vi "LabVIEW Measurement UI - Open & Run.vi"(8 "error in":errorcluster, 10 "UI Subpanel":refnum<vi>, 11 "Measurement Client Wrapper in":refnum<class "Measurement Client Wrapper.lvclass">) -> (0 "error out":errorcluster, 2 "Valid UI?":bool, 3 "Measurement Client Wrapper":refnum<class "Measurement Client Wrapper.lvclass">)   [LabVIEW 2020, in "Measurement Client Wrapper.lvclass"]
uses:
  Measurement Client Wrapper.lvclass
  Measurement Client Wrapper.lvclass/Measurement Client Wrapper.ctl
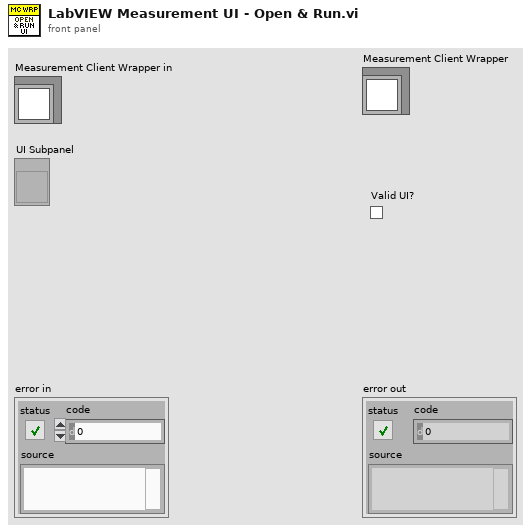
[diagram p1: front panel]
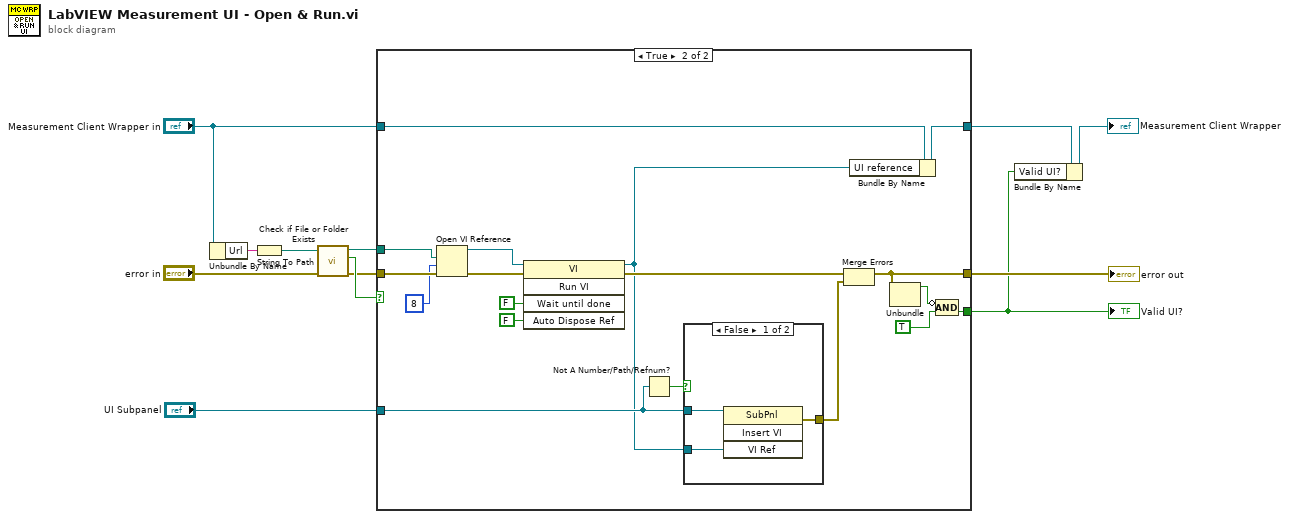
[diagram p0: block diagram]
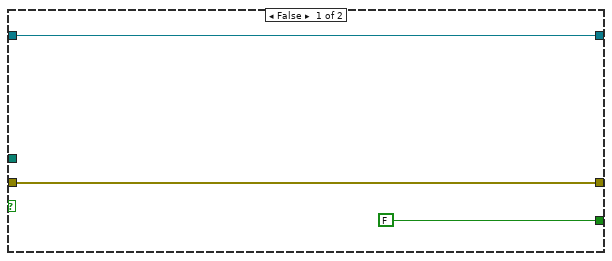
[diagram p2: hidden frame]
diagram:
  n1 = Unbundle By Name("Measurement Client Wrapper in") -> ("Url"=w5:string)
  n2 = String To Path(string=w5) -> (path=w4:path)
  n3 = call <vilib>:"Check if File or Folder Exists.vi"("error in (no error)"="error in", "path"=w4) -> ("error out"=w10:errorcluster, "file or folder exists?"=w11:bool, "dup path"=w9:path)  [unwired: 7 in]
  n4 = case shown="True" w11 {
    tunnel: w10 -> [w15 w33]
    tunnel: w9 -> [_ w32]
    tunnel: [w15 w17] -> w8
    tunnel: [FALSE w25] -> w2
    tunnel: "Measurement Client Wrapper in" -> [w13 w23]
    tunnel: [w13 w22] -> w3
    tunnel: "UI Subpanel" -> [_ w20]
    frame False {
    }
    frame True {
      n5 = Open VI Reference(vi path=w32, options=8, error in (no error)=w33) -> (vi reference=w29:refnum<vi>, error out=w30:errorcluster)  [unwired: 3 in]
      n6 = invoke class="VI" method="Run VI"(reference=w29, error in=w30, "Wait until done"=FALSE ("Wait Until Done"), "Auto Dispose Ref"=FALSE ("Auto Dispose Reference")) -> (reference out=w18:refnum<vi>, error out=w19:errorcluster)  [unwired: 1 in, 3 out]
      n7 = Not A Number/Path/Refnum?(number/path/refnum=w20) -> (NaN/Path/Refnum?=w21:bool)
      n8 = case shown="False" w21 {
        tunnel: w20 -> [w36 _]
        tunnel: w18 -> [w35 _]
        tunnel: [w34 _] -> w16
        frame False {
          n9 = invoke class="SubPnl" method="Insert VI"(reference=w36, "VI Ref"=w35) -> (error out=w34:errorcluster)  [unwired: 2 in, 3 out]
        }
        frame True {
        }
      }
      n10 = Merge Errors(w19, w16) -> (w17:errorcluster)
      n11 = Bundle By Name(cluster=w23, "UI reference"=w18) -> (w22:refnum<class "Measurement Client Wrapper.lvclass">)
      n12 = Unbundle(w17) -> ("status"=w24:bool)  [unwired: 2 out]
      n13 = Compound Arithmetic op=AND(invert w24, TRUE) -> (w25:bool)
    }
  }
  "error out" <- w8
  "Valid UI?" <- w2
  n14 = Bundle By Name(cluster=w3, "Valid UI?"=w2) -> (→"Measurement Client Wrapper":refnum<class "Measurement Client Wrapper.lvclass">)
